vi "Configure Current Limit.vi"(0 "VISA resource name":refnum<visa-resource-name>, 2 "Communication Address (0)":i16 max=254 format="%x", 7 "Current Limit (0)":dbl min=0.0 max=6.0 format="%#.2g", 11 "error in (no error)":errorcluster) -> (4 "VISA resource name out":refnum<visa-resource-name>, 15 "error out":errorcluster)   [LabVIEW 2019, in "BK Precision 178XB Series.lvlib"]
doc: "This VI configures the current limiting value. The power supply will trip over to CC (Constant Current) mode if the amount of current drawn by a device connected to the supply exceeds this value."
uses:
  BK Precision 178XB Series.lvlib
panel:
  # "(c) 2009 B&K PRECISION CORPORATION.  ALL RIGHTS RESERVED."
  # "A"
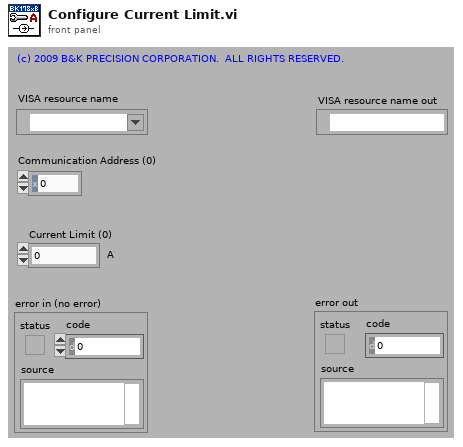
[diagram p1: front panel]
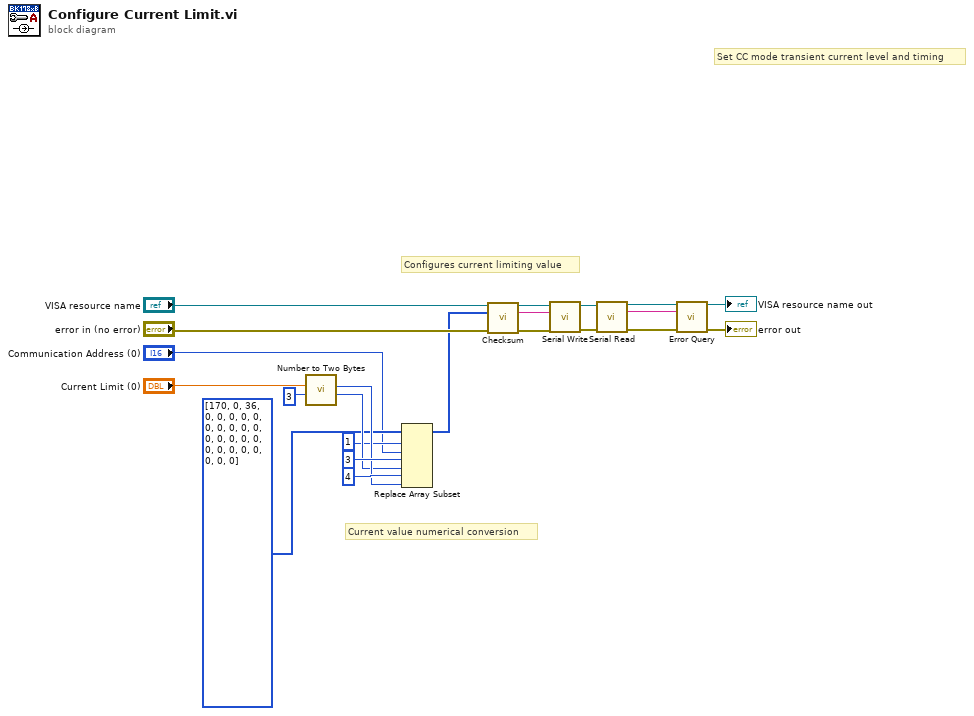
[diagram p0: block diagram]
diagram:
  # "Configures current limiting value"
  # "Current value numerical conversion"
  # "Set CC mode transient current level and timing"
  n1 = call "Number to Two Bytes.vi"("Fractional Precision (0)"=3, "Input Value (0)"="Current Limit (0)") -> ("Byte 2"=w12:i32, "Byte 1"=w13:i32)  [unwired: 8 in]
  n2 = Replace Array Subset(array=i16[] [170, 0, 36, 0, 0, 0, 0, 0, 0, 0, 0, 0, 0, 0, 0, 0, 0, 0, 0, 0, 0, 0, 0, 0, 0, 0], new element #1="Communication Address (0)", index #1=1, new element #2=w12, index #2=3 ("index"), new element #3=w13, index #3=4 ("index")) -> (w9:i16[])
  n3 = call "Checksum.vi"("VISA resource name"="VISA resource name", "Command Frame Array"=w9, "error in (no error)"="error in (no error)") -> ("VISA resource name out"=w17:refnum<visa-resource-name>, "Output String"=w8:string, "error out"=w18:errorcluster)  [unwired: 8 in, 2 out]
  n4 = call "Serial Write.vi"("error in (no error)"=w18, "Input Command Frame"=w8, "VISA resource name"=w17) -> ("error out"=w19:errorcluster, "VISA resource name out"=w20:refnum<visa-resource-name>)  [unwired: 6 in, 1 out]
  n5 = call "Serial Read.vi"("error in (no error)"=w19, "VISA resource name"=w20) -> ("error out"=w6:errorcluster, "Read Buffer"=w5:string, "VISA resource name out"=w7:refnum<visa-resource-name>)  [unwired: 7 in]
  n6 = call "Error Query.vi"("VISA resource name"=w7, "Input Read Buffer 1"=w5, "error in (no error)"=w6) -> ("VISA resource name out"=→"VISA resource name out":refnum<visa-resource-name>, "error out"=→"error out":errorcluster)  [unwired: 7 in, 4 out]
